vi "Flush Data Tick Counter.vi"(7 "Reset":bool, 11 "Increment":bool) -> (3 "Periods":u16)   [LabVIEW 2014]
panel:
  # "Copyright 2014 Vidrio Technologies\nScanImage 5 software is licensed under the Apache License, Version 2.0 (the \"License\"); you may not use any files contained\nwithin the ScanImage 5 release except in compliance with the License. You may obtain a copy of the License at\n http://www.apache.org/licenses/LICENSE-2.0\nUnless required by applicable law or agreed to in writing, software distributed under the License is distributed on an\n\"AS IS\" BASIS, WITHOUT WARRANTIES OR CONDITIONS OF ANY KIND, either express or implied. See the License for the\n specific language governing permissions and limitations under the License."
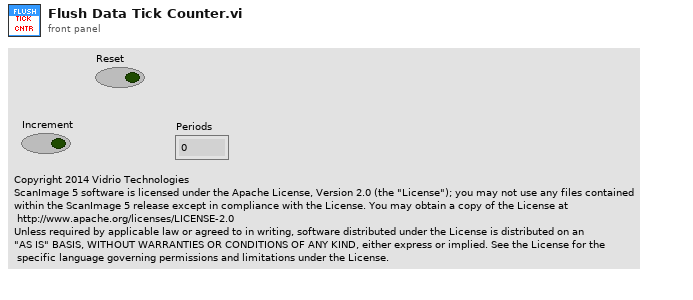
[diagram p1: front panel]
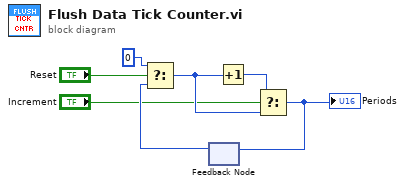
[diagram p0: block diagram]
diagram:
  n1 = feedback #1() -> (w5:u16)  [unwired: 1 in]
  n2 = Select(t=u16 0, s="Reset", f=w5) -> (s? t:f=w6:u16)
  n3 = Increment(x=w6) -> (x+1=w1:u16)
  n4 = Select(t=w1, s="Increment", f=w6) -> (s? t:f=w7:u16)
  "Periods" <- w7
  n5 = feedback-in #1(w7) -> ()
